vi "Update Hardware Settings.vi"(0 "Queue in":refnum<queue>, 1 "Serial Numbers Ref":refnum<vi>, 5 "Hardware Settings in":T3, 7 "OldVal":T1, 9 "NewVal":T1, 11 "error in (no error)":errorcluster) -> (4 "Queue out":refnum<queue>, 6 "Channel Config":T2[](array[typedef]), 8 "Hardware Settings out":T3, 10 "Serial Numbers":string[](array[string]), 14 "Serial Number Header?":bool, 15 "error out":errorcluster)   [LabVIEW 2026, in "Settings.lvlib"]
uses:
  Settings.lvlib
  Acquisition/Hardware Configuration.ctl
  Acquisition/Hardware Cluster Configuration.ctl
  support/Architecture/Message Queue/Message Cluster.ctl
  controls/UI/UUT Channel Config.ctl
  controls/UI/UUT Channels Config.ctl
  controls/Messaging Payloads/MSG FetchSensorID Payload.ctl
  Acquisition/Acquisition.lvlib
  support/Architecture/Message Queue/Message Queue.lvlib
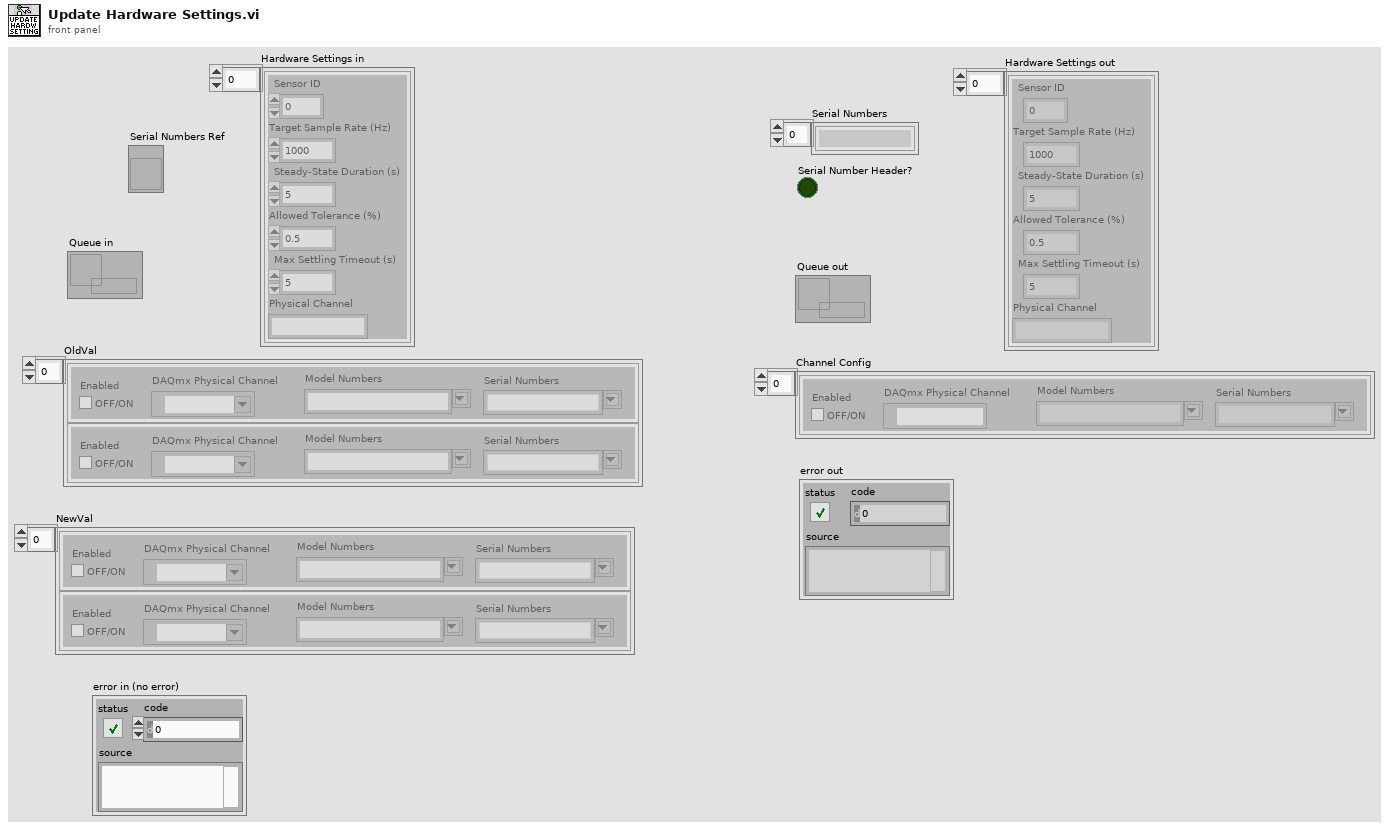
[diagram p1: front panel]
types:
  T1 = typedef "UUT Channels Config.ctl" = T2[]
  T2 = typedef "UUT Channel Config.ctl" = cluster{"DAQmx Physical Channel":tag, "Serial Numbers":string, "Enabled":bool, "Model Numbers":string}
  T3 = typedef "Acquisition.lvlib/Hardware Configuration.ctl" = T4[]
  T4 = typedef "Acquisition.lvlib/Hardware Cluster Configuration.ctl" = cluster{"Sensor ID":i32, "Target Sample Rate (Hz)":dbl, "Steady-State Duration (s)":i32, "Allowed Tolerance (%)":dbl, "Max Settling Timeout (s)":i32, "Physical Channel":string}
  T5 = typedef "MSG FetchSensorID Payload.ctl" = cluster{"SensorID":i32, "Serial Number":string, "Model Number":string}
  T6 = typedef "MSG FetchConfiguration Payload.ctl" = cluster{"Serial Numbers":string[], "Hardware Settings Cluster":T4}
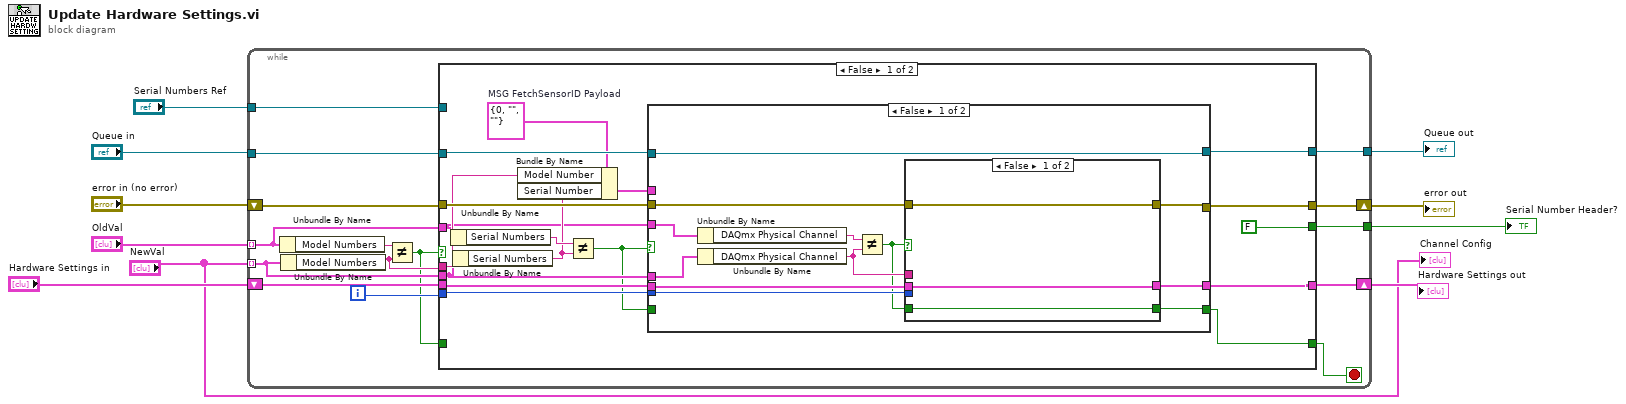
[diagram p0: block diagram]
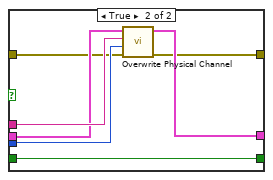
[diagram p2: hidden frame]
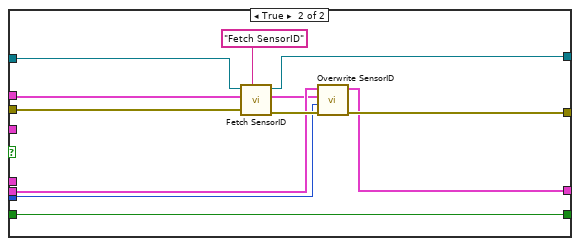
[diagram p3: hidden frame]
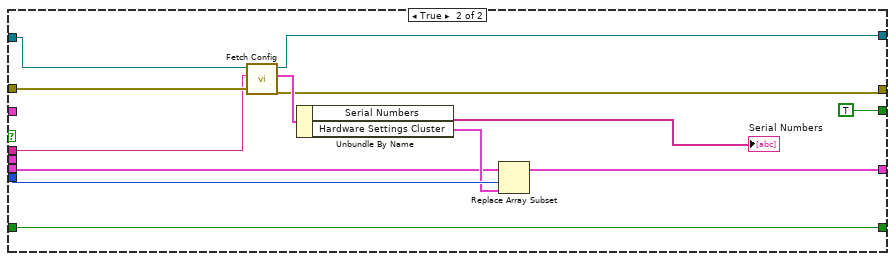
[diagram p4: hidden frame]
diagram:
  n1 = while {
    tunnel: "OldVal" -> [w23] mode=indexing
    tunnel: "NewVal" -> [w16] mode=indexing
    tunnel: "Queue in" -> [w25]
    shift-right: [w22] -> w6
    shift-left: "error in (no error)" -> [w21]
    tunnel: [w20] -> w8
    shift-right: [w19] -> w9
    shift-left: "Hardware Settings in" -> [w17]
    tunnel: "Serial Numbers Ref" -> [w14]
    tunnel: [w13] -> w1
    i -> [w18]
    stop <- w11 stop-if-true
    n2 = Unbundle By Name(w23) -> ("Model Numbers"=w24:string)
    n3 = Unbundle By Name(w16) -> ("Model Numbers"=w15:string)
    n4 = Not Equal?(x=w24, y=w15) -> (x != y?=w12:bool)
    n5 = case shown="False" w12 {
      tunnel: w25 -> [w41 w89]
      tunnel: w23 -> [w30 _]
      tunnel: [w36 w81] -> w19
      tunnel: w21 -> [w40 w88]
      tunnel: [w35 w79] -> w22
      tunnel: [w39 w86] -> w20
      tunnel: w18 -> [w38 w85]
      tunnel: w17 -> [w37 w83]
      tunnel: w16 -> [w29 _]
      tunnel: w15 -> [w32 w82]
      tunnel: w14 -> [_ _]
      tunnel: [FALSE TRUE] -> w13
      tunnel: [w26 w77] -> w11
      tunnel: w12 -> [_ w77]
      frame False {
        w34 = T5 {"SensorID"=0, "Serial Number"="", "Model Number"=""}  # MSG FetchSensorID Payload
        n6 = Unbundle By Name(w30) -> ("Serial Numbers"=w42:string)
        n7 = Unbundle By Name(w29) -> ("Serial Numbers"=w31:string)
        n8 = Bundle By Name(cluster=w34, "Model Number"=w32, "Serial Number"=w31) -> (w33:T5)
        n9 = Not Equal?(x=w42, y=w31) -> (x != y?=w27:bool)
        n10 = case shown="False" w27 {
          tunnel: w41 -> [w45 w76]
          tunnel: w40 -> [w47 w75]
          tunnel: [w46 w71] -> w35
          tunnel: [w45 w73] -> w39
          tunnel: w38 -> [w50 w70]
          tunnel: w37 -> [w49 w69]
          tunnel: [w48 w68] -> w36
          tunnel: w33 -> [_ w66]
          tunnel: w30 -> [w53 _]
          tunnel: w29 -> [w52 _]
          tunnel: w27 -> [_ w65]
          tunnel: [w44 w65] -> w26
          frame False {
            n11 = Unbundle By Name(w53) -> ("DAQmx Physical Channel"=w54:tag)
            n12 = Unbundle By Name(w52) -> ("DAQmx Physical Channel"=w51:tag)
            n13 = Not Equal?(x=w54, y=w51) -> (x != y?=w43:bool)
            n14 = case shown="False" w43 {
              tunnel: w51 -> [_ w63]
              tunnel: w50 -> [_ w64]
              tunnel: w49 -> [w56 w62]
              tunnel: [w56 w61] -> w48
              tunnel: w47 -> [w57 w60]
              tunnel: [w57 w59] -> w46
              tunnel: w43 -> [w55 w58]
              tunnel: [w55 w58] -> w44
              frame False {
              }
              frame True {
                n15 = call "Overwrite Physical Channel.vi"("error in (no error)"=w60, "Index"=w64, "DAQmx Physical Channel"=w63, "Hardware Settings in"=w62) -> ("error out"=w59:errorcluster, "Hardware Settings out"=w61:T3)  [unwired: 6 in]
              }
            }
          }
          frame True {
            n16 = call "Fetch SensorID.vi"("Message"="Fetch SensorID", "error in (no error)"=w75, "MSG FetchSensorID Payload in"=w66, "Database in"=w76) -> ("error out"=w72:errorcluster, "MSG FetchSensorID Payload out"=w67:T5, "Database out"=w73:refnum<queue>)  [unwired: 5 in]
            n17 = call "Overwrite SensorID.vi"("error in (no error)"=w72, "Index"=w70, "MSG FetchSensorID Payload"=w67, "Hardware Settings in"=w69) -> ("error out"=w71:errorcluster, "Hardware Settings out"=w68:T3)  [unwired: 6 in]
          }
        }
      }
      frame True {
        n18 = call "Fetch Config.vi"("error in (no error)"=w88, "ModelNumber"=w82, "Database in"=w89) -> ("error out"=w79:errorcluster, "Model Details Payload"=w87:T6, "Database out"=w86:refnum<queue>)  [unwired: 6 in]
        n19 = Unbundle By Name(w87) -> ("Serial Numbers"=→"Serial Numbers":string[], "Hardware Settings Cluster"=w84:T4)
        n20 = Replace Array Subset(array=w83, new element=w84, index=w85) -> (w81:T3)
      }
    }
  }
  "Hardware Settings out" <- w9
  "Queue out" <- w8
  "error out" <- w6
  "Serial Number Header?" <- w1
  "Channel Config" <- "NewVal"
